vi "ReadWindVaneData.vi"(8 "Error in":errorcluster, 11 "Wind Vane Queue Cluster":T1) -> (0 "error out":errorcluster, 3 "Measured wind angle":dbl)   [LabVIEW 2013]
doc: "This VI takes in wind sensor data from whichever wind sensor is being used and writes it to the proper queues. Needs to be calibrated with whatever wind sensors we choose.\n\nEric Schneider, March 2014"
uses:
  <vilib>/measure/NI_MAPro.lvlib
  <vilib>/measure/mascope.llb/Pulse Measurements 1 chan.vi
  Data/TypeDefs/WindData Queue Cluster.ctl
panel:
  out "pulse duration":dbl format="%.2g"
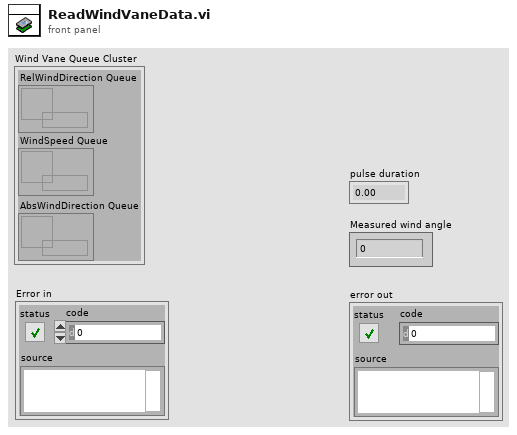
[diagram p1: front panel]
types:
  T1 = typedef "WindData Queue Cluster.ctl" = cluster{"RelWindDirection Queue":refnum<queue>, "WindSpeed Queue":refnum<queue>, "AbsWindDirection Queue":refnum<queue>}
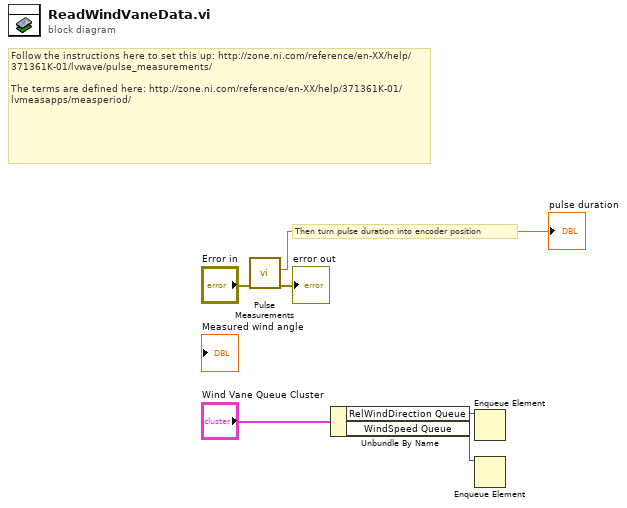
[diagram p0: block diagram]
diagram:
  # "Then turn pulse duration into encoder position"
  # "Follow the instructions here to set this up: http://zone.ni.com/reference/en-XX/help/371361K-01/lvwave/pulse_measurements/\n\nThe terms are defined here: http://zone.ni.com/reference/en-XX/help/371361K-01/lvmeasapps/measperiod/"
  n1 = call-poly <vilib>:"Pulse Measurements.vi"("error in (no error)"="Error in") -> ("error out"=→"error out":errorcluster, "pulse duration"=→"pulse duration":dbl)  [unwired: 6 in, 3 out]
  n2 = Unbundle By Name("Wind Vane Queue Cluster") -> ("RelWindDirection Queue"=w2:refnum<queue>, "WindSpeed Queue"=w1:refnum<queue>)
  n3 = Enqueue Element(queue=w2) -> ()  [unwired: 3 in, 3 out]
  n4 = Enqueue Element(queue=w1) -> ()  [unwired: 3 in, 3 out]
